vi "lockin parameters header.vi"() -> (0 "Array":string[][](array[string]))   [LabVIEW 2021]
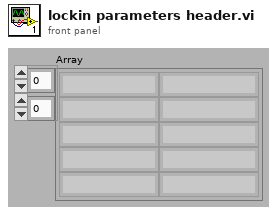
[diagram p1: front panel]
types:
  T1 = enum16{"Set Amplitude", "Get Amplitude", "Set Frequency", "Get Frequency", "Set Harmonic", "Get Harmonic", "Set Phase", "Get Phase", "Auto Phase", "Add to Phase", "Autogain", "Set Time Constant", "Get Time Constant", "Set Sensitivity", "Get Sensitivity", "Set Input A", "Set Input A-B", "Get Input Setting", "Set Offset", "Get Offset"}
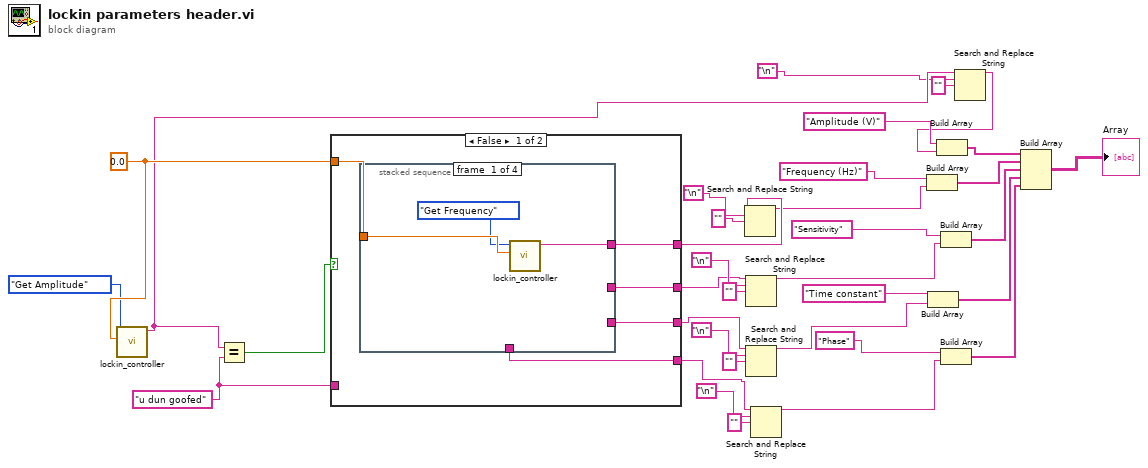
[diagram p0: block diagram]
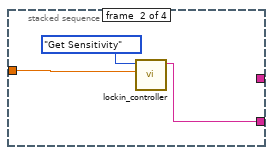
[diagram p2: hidden frame]
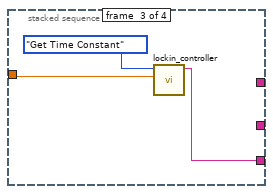
[diagram p3: hidden frame]
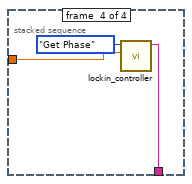
[diagram p4: hidden frame]
diagram:
  w21 = "u dun goofed"
  w24 = 0.0 ("Numerical Argument")
  n1 = call "lockin_controller.vi"("Numerical Argument"=w24, "Command"=T1."Get Amplitude") -> ("Response"=w20:string)  [unwired: 9 in]
  n2 = Equal?(x=w20, y=w21) -> (x = y?=w22:bool)
  n3 = case shown="False" w22 {
    tunnel: w24 -> [w40 _]
    tunnel: [w39 w53] -> w14
    tunnel: [w38 w53] -> w6
    tunnel: [w37 w53] -> w4
    tunnel: [w36 w53] -> w2
    tunnel: w21 -> [_ w53]
    frame False {
      n4 = stacked-sequence {
        tunnel: w40 -> [w43 w46 w49 w51]
        tunnel: [w41 _ _ _] -> w39
        tunnel: [_ w44 _ _] -> w38
        tunnel: [_ _ w47 _] -> w37
        tunnel: [_ _ _ w52] -> w36
        frame #0 {
          n5 = call "lockin_controller.vi"("Numerical Argument"=w43, "Command"=T1."Get Frequency") -> ("Response"=w41:string)  [unwired: 9 in]
        }
        frame #1 {
          n6 = call "lockin_controller.vi"("Numerical Argument"=w46, "Command"=T1."Get Sensitivity") -> ("Response"=w44:string)  [unwired: 9 in]
        }
        frame #2 {
          n7 = call "lockin_controller.vi"("Numerical Argument"=w49, "Command"=T1."Get Time Constant") -> ("Response"=w47:string)  [unwired: 9 in]
        }
        frame #3 {
          n8 = call "lockin_controller.vi"("Numerical Argument"=w51, "Command"=T1."Get Phase") -> ("Response"=w52:string)  [unwired: 9 in]
        }
      }
    }
    frame True {
    }
  }
  n9 = Search and Replace String(input string=w14, search string="\n", replace string="" ("replace string (\"\")")) -> (result string=w13:string)  [unwired: 5 in, 3 out]
  n10 = Search and Replace String(input string=w6, search string="\n", replace string="" ("replace string (\"\")")) -> (result string=w5:string)  [unwired: 5 in, 3 out]
  n11 = Search and Replace String(input string=w4, search string="\n", replace string="" ("replace string (\"\")")) -> (result string=w3:string)  [unwired: 5 in, 3 out]
  n12 = Search and Replace String(input string=w2, search string="\n", replace string="" ("replace string (\"\")")) -> (result string=w1:string)  [unwired: 5 in, 3 out]
  n13 = Build Array("Frequency (Hz)", w13) -> (w28:string[])
  n14 = Build Array("Time constant", w3) -> (w26:string[])
  n15 = Build Array("Sensitivity", w5) -> (w27:string[])
  n16 = Build Array("Phase", w1) -> (w25:string[])
  n17 = Search and Replace String(input string=w20, search string="\n", replace string="" ("replace string (\"\")")) -> (result string=w19:string)  [unwired: 5 in, 3 out]
  n18 = Build Array("Amplitude (V)", w19) -> (w34:string[])
  n19 = Build Array(w34, w28, w27, w26, w25) -> (→"Array":string[][])
